vi "Car wash assignment.vi"() -> ()   [LabVIEW 2019]
panel:
  in  "Under Body Wash Position Switch":bool
  in  "Air Dry Position Switch":bool
  in  "Main Wash Position Switch":bool
  out "Wash Select":string
  out "Main wash TimeRemaining":dbl
  out "Main wash TimeElapsed":dbl
  out "Main wash":dbl
  out "Under/Air TimeRemaining":dbl
  out "Under/ Air TimeElapsed":dbl
  out "Under/Air":dbl
  in  "STOP":bool
  out "Vehicle Out of Position/\nPause":bool
  out "Air Dry":bool
  out "Clear Water Rinse":bool
  out "Main High Pressure Wash":bool
  out "Soap Application":bool
  out "Under Body Wash":bool
  in  "Economy Wash":bool
  in  "Deluxe Wash":bool
  out "Last Process":bool
  # "Purchase Selection"
  # "Car Wash Indicators"
  # "Car Wash Simulation Switches"
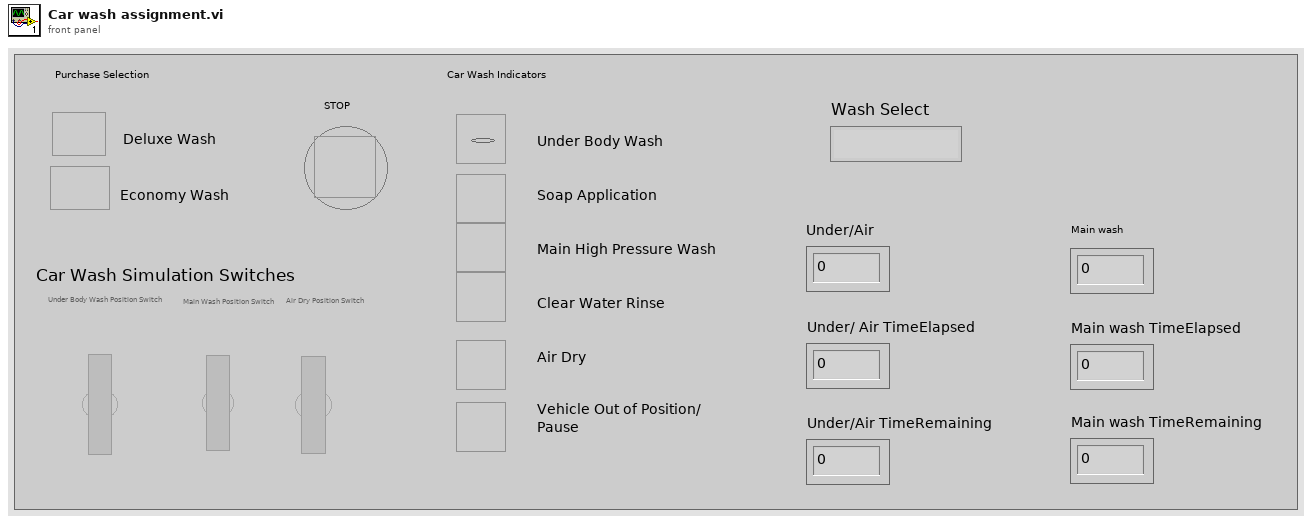
[diagram p1: front panel]
types:
  T1 = enum16{"Soap Application", "Pressure Wash", "CLear water rinse", "Vehicle out"}
  T2 = enum16{"Under Body Wash", "Soap Application", "Pressure Wash", "Clear Water Rinse", "Air Dry", "Vehicle out"}
  T3 = enum8{"Enabled", "Disabled", "Disabled and Grayed Out"}
  T4 = enum16{"Soap Application", "Pressure Wash", "Clear water rinse", "Vehicle out"}
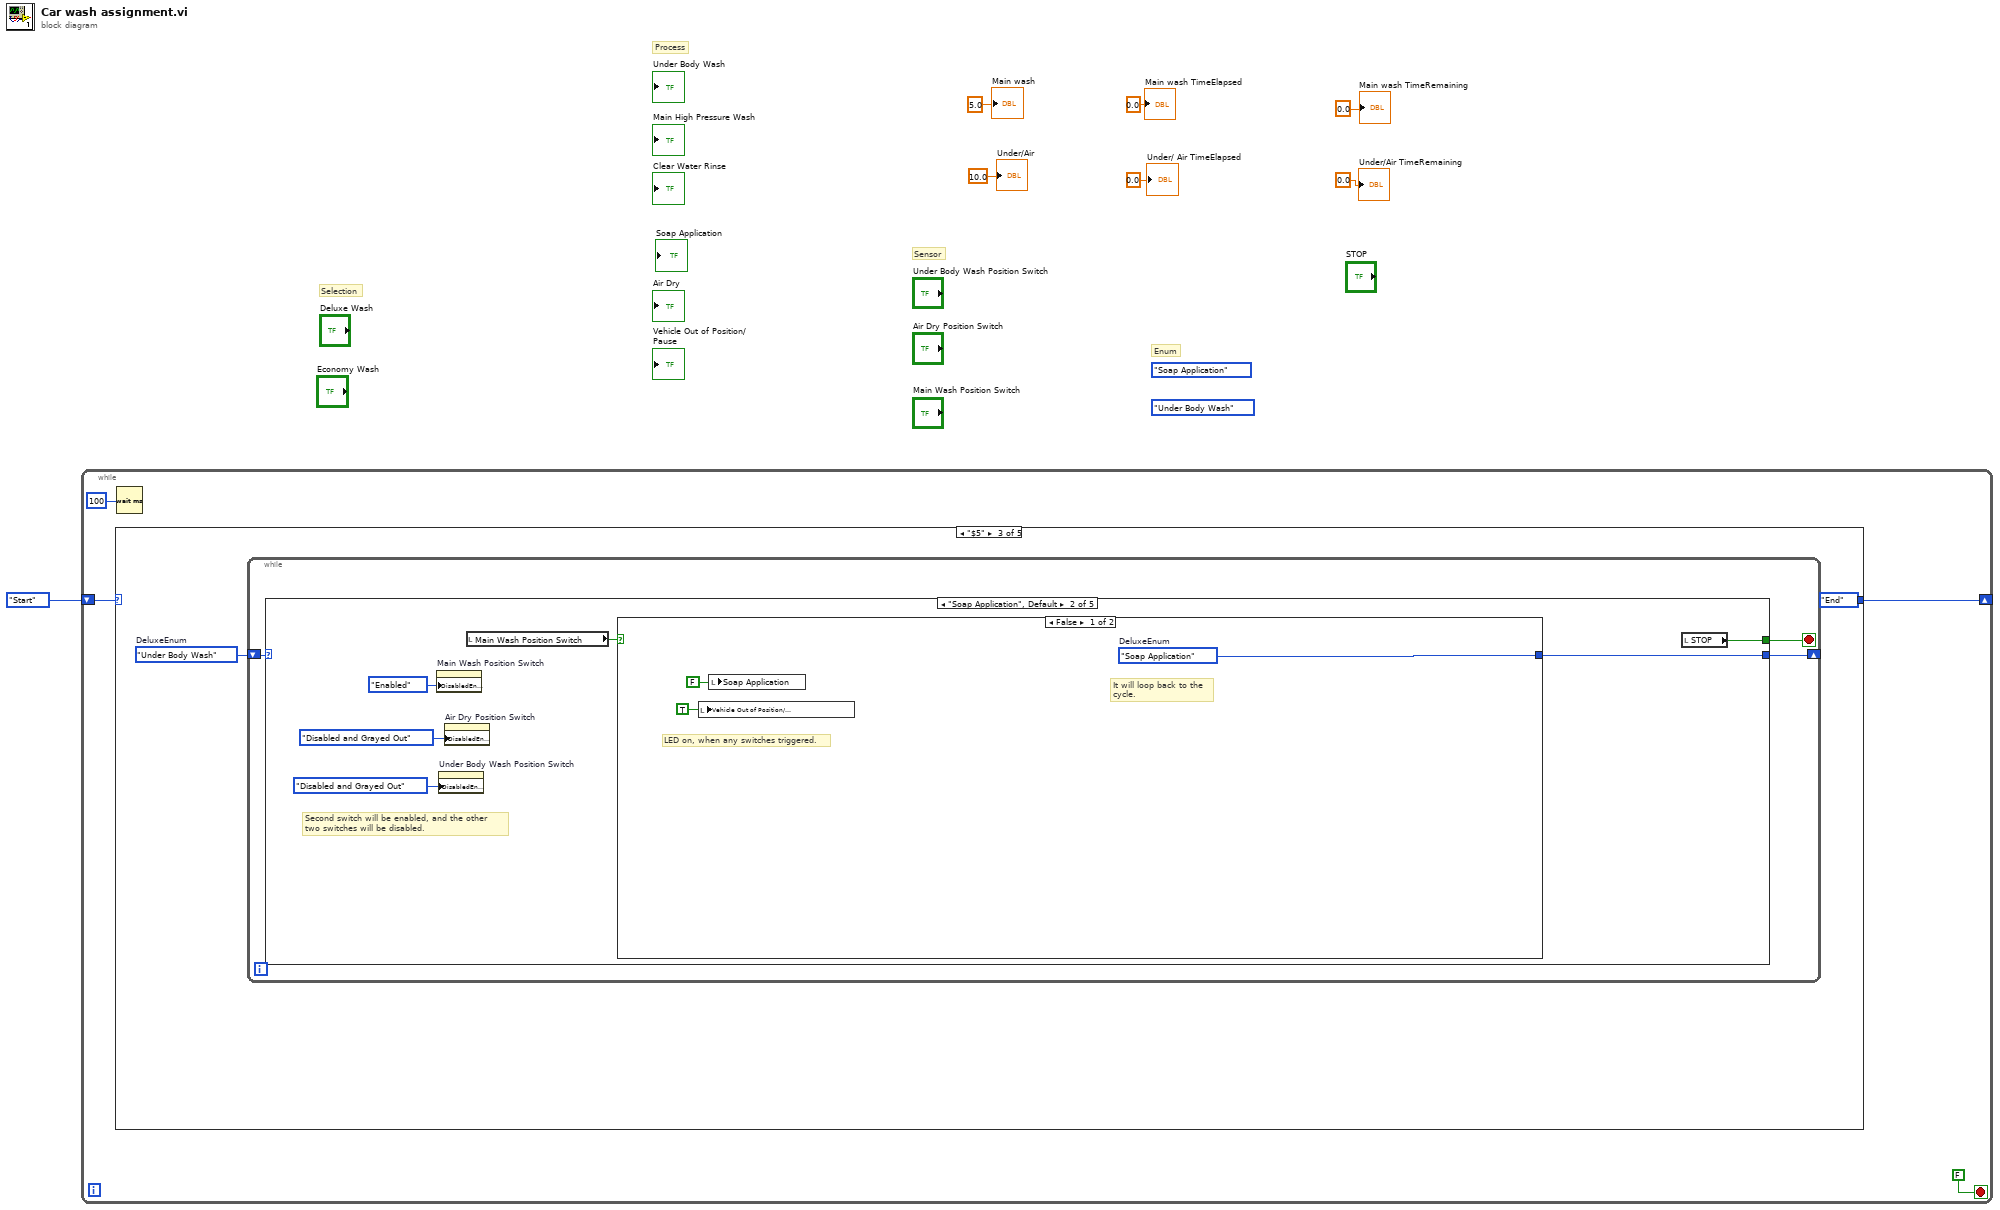
[diagram p0: block diagram]
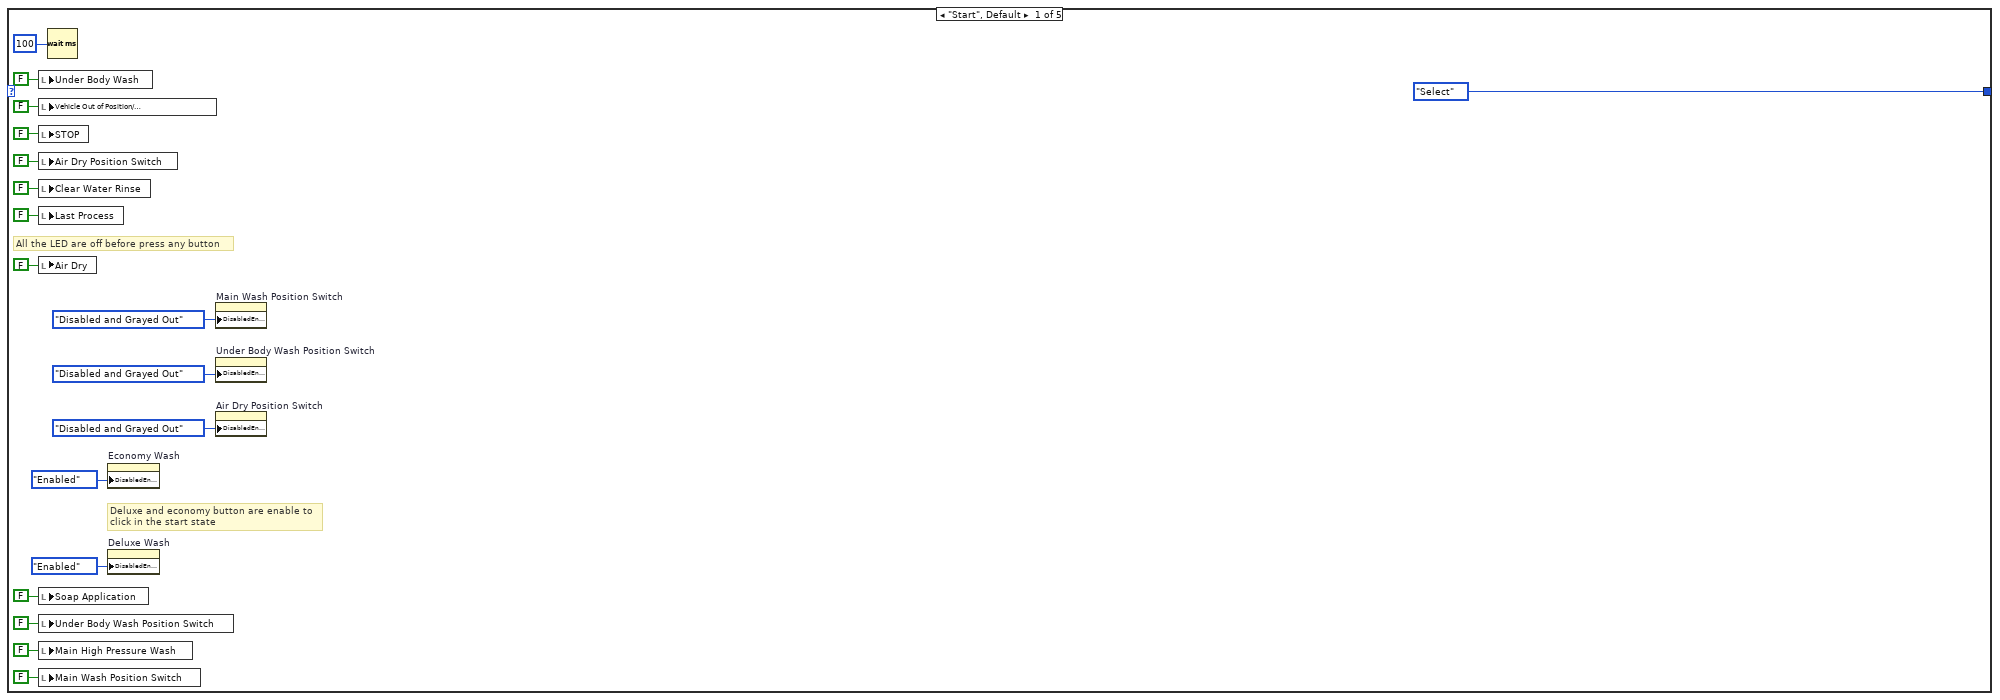
[diagram p2: hidden frame]
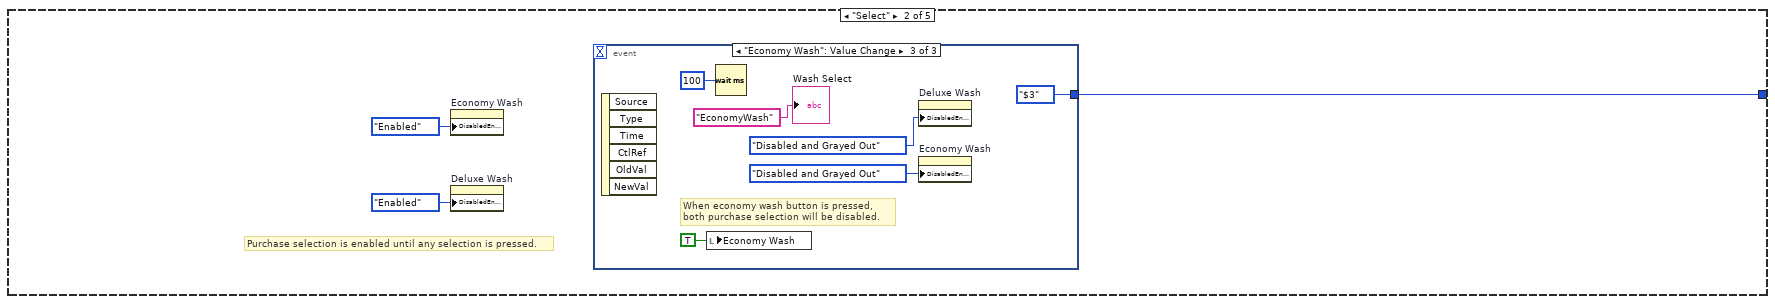
[diagram p3: hidden frame]
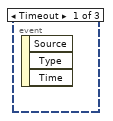
[diagram p4: hidden frame]
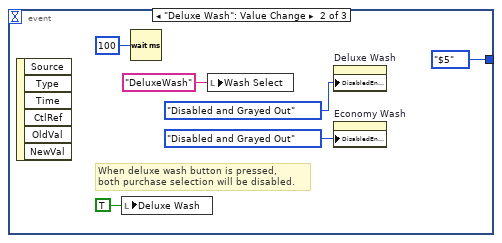
[diagram p5: hidden frame]
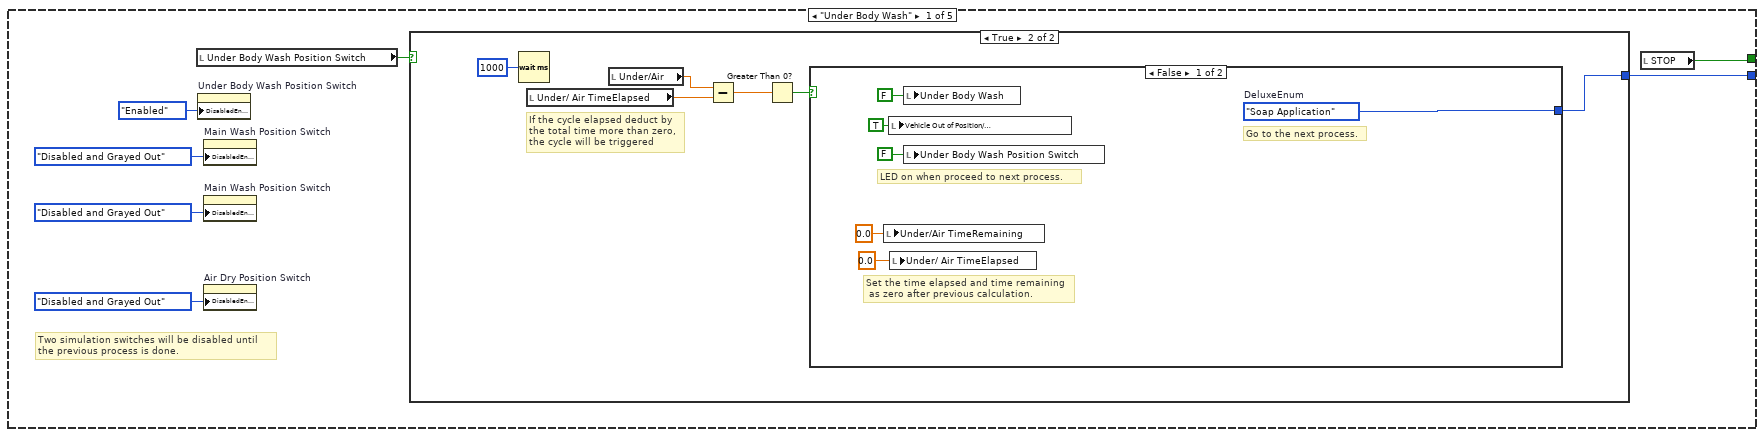
[diagram p6: hidden frame]
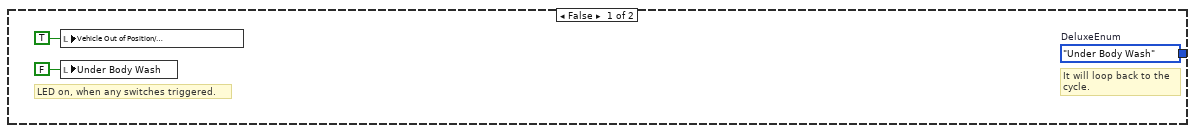
[diagram p7: hidden frame]
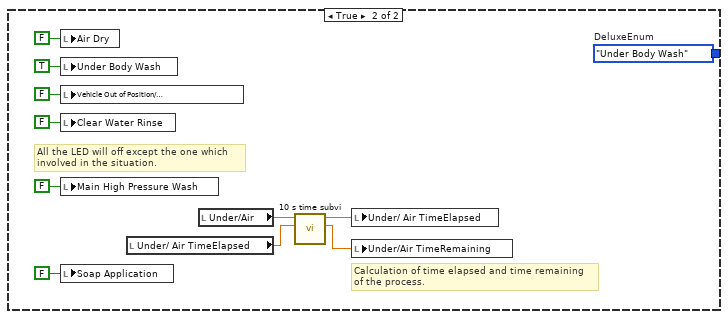
[diagram p8: hidden frame]
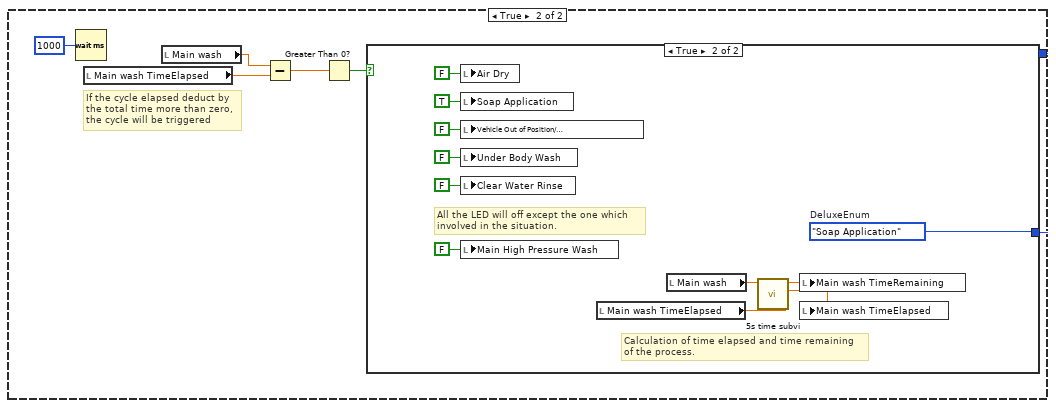
[diagram p9: hidden frame]
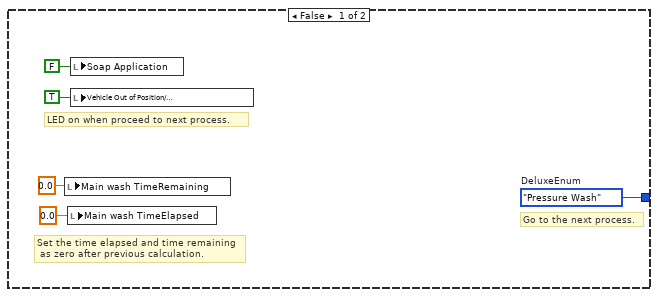
[diagram p10: hidden frame]
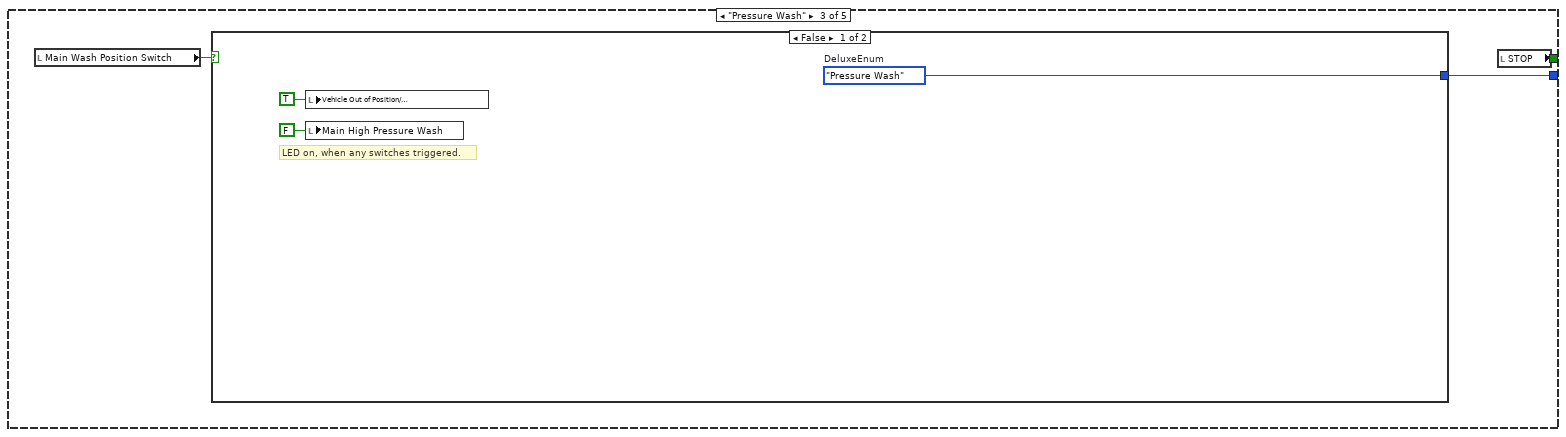
[diagram p11: hidden frame]
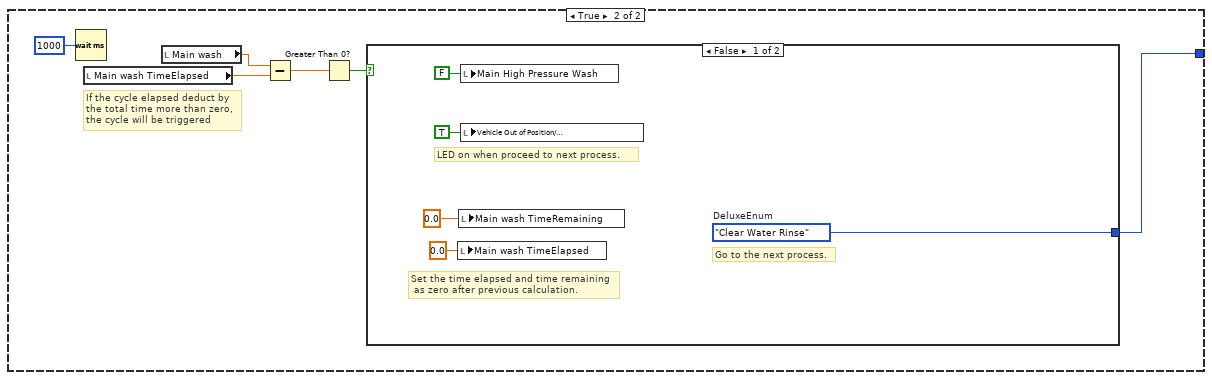
[diagram p12: hidden frame]
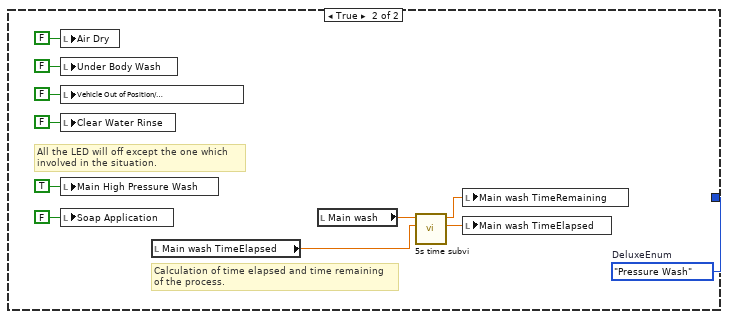
[diagram p13: hidden frame]
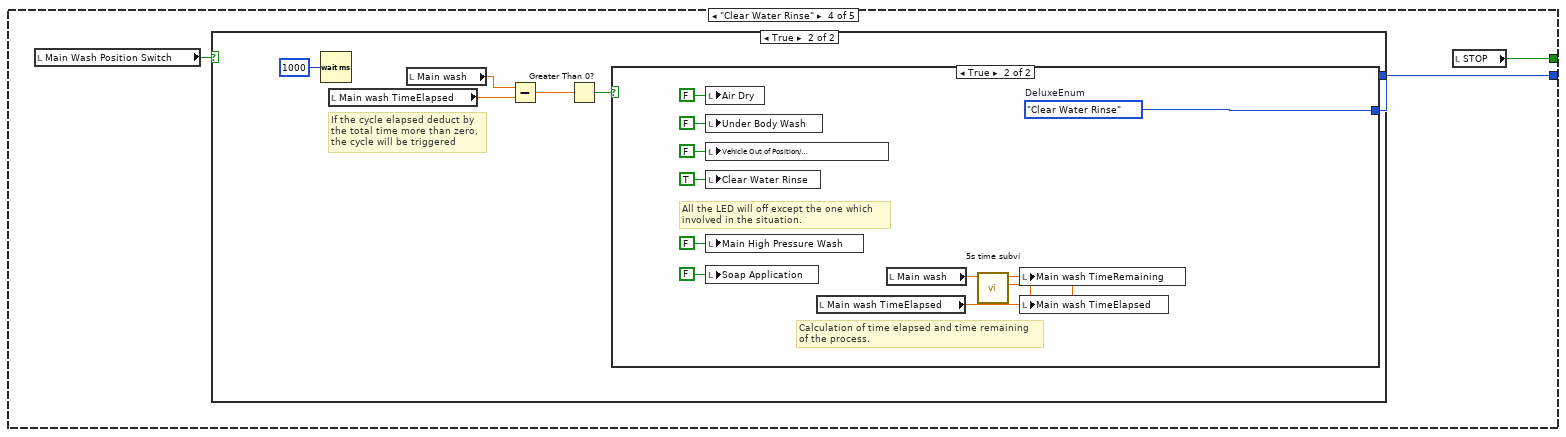
[diagram p14: hidden frame]
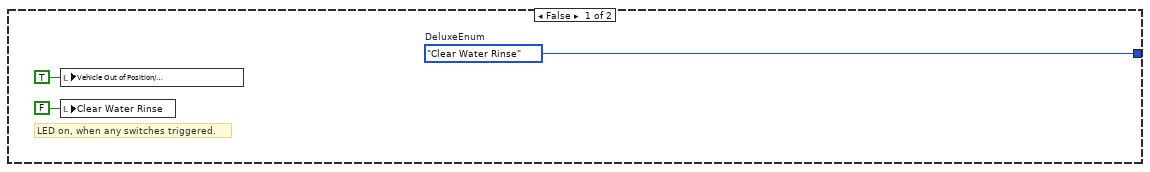
[diagram p15: hidden frame]
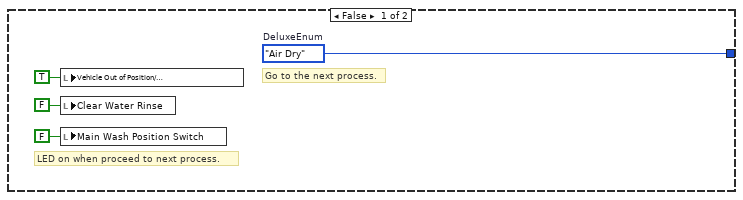
[diagram p16: hidden frame]
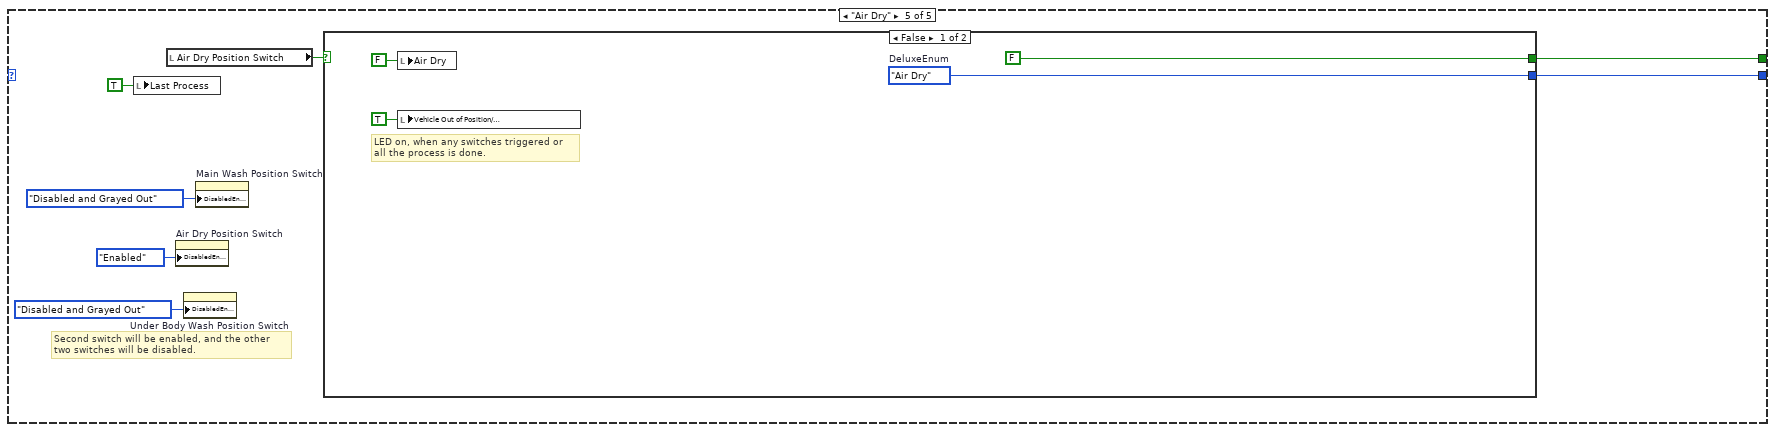
[diagram p17: hidden frame]
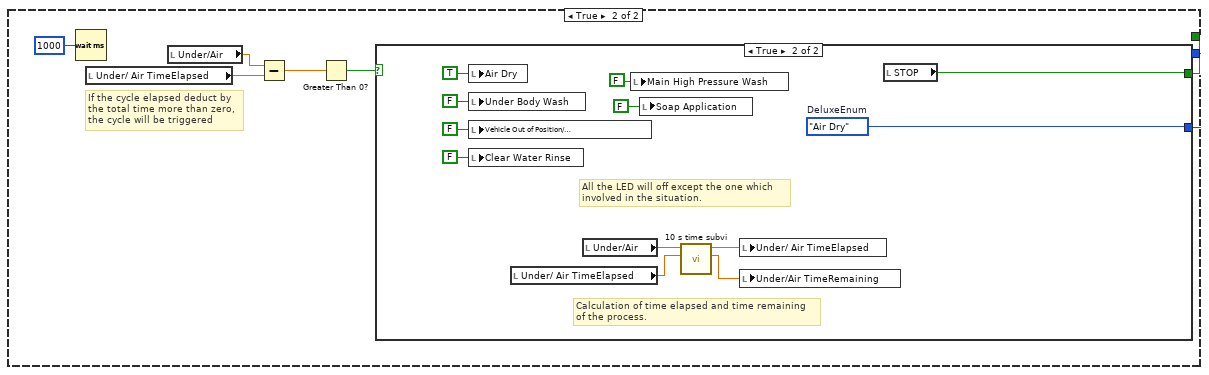
[diagram p18: hidden frame]
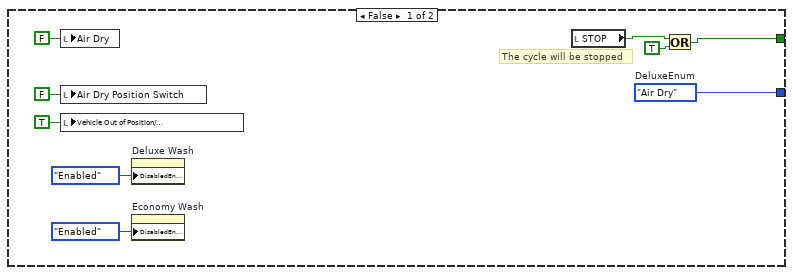
[diagram p19: hidden frame]
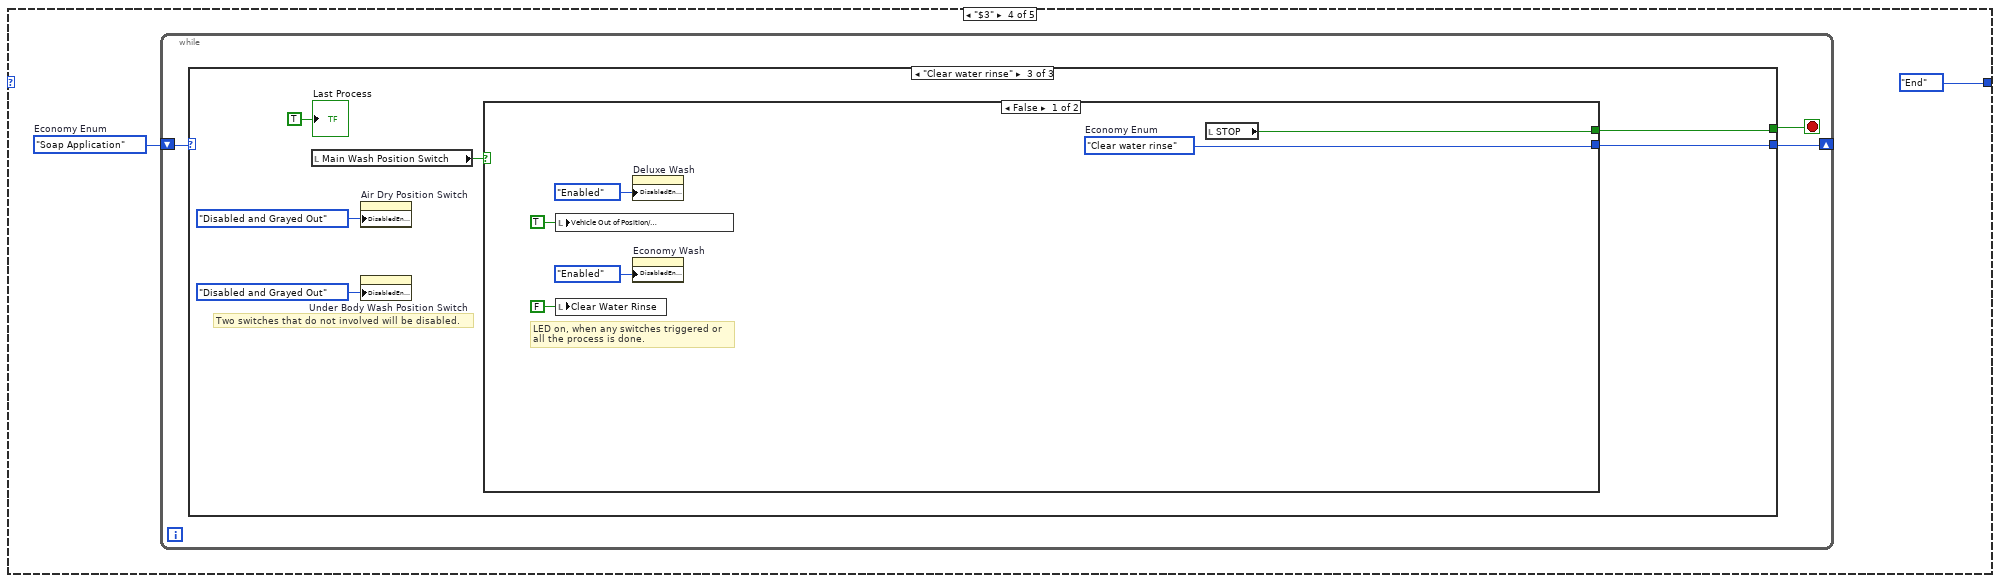
[diagram p20: hidden frame]
diagram:
  (unwired) T1."Soap Application" ("Economy Enum")
  (unwired) T2."Under Body Wash" ("Enum")
  # "Enum"
  # "Process"
  # "Sensor"
  # "Selection"
  n1 = while {
    shift-right: [w10] -> _
    shift-left: enum16{"Start", "Select", "$5", "$3", "End"}."Start" -> [w11]
    stop <- FALSE stop-if-true
    n2 = case shown="\"$5\"" w11 {
      tunnel: [enum16{"Start", "Select", "$5", "$3", "End"}."Select" w32 enum16{"Start", "Select", "$5", "$3", "End"}."End" enum16{"Start", "Select", "$5", "$3", "End"}."End" enum16{"Start", "Select", "$5", "$3", "End"}."Start"] -> w10
      frame "Start", Default {
        # "All the LED are off before press any button"
        # "Deluxe and economy button are enable to\nclick in the start state"
        n3 = local write "Under Body Wash"(FALSE ("Under Body Wash")) -> ()
        n4 = local write "Vehicle Out of Position/\nPause"(FALSE ("Vehicle Out of Position/\nPause")) -> ()
        n5 = local write "STOP"(FALSE ("STOP")) -> ()
        n6 = local write "Air Dry Position Switch"(FALSE ("Air Dry Position Switch")) -> ()
        n7 = local write "Clear Water Rinse"(FALSE ("Clear Water Rinse")) -> ()
        n8 = local write "Last Process"(FALSE ("Last Process")) -> ()
        n9 = local write "Air Dry"(FALSE ("Air Dry")) -> ()
        n10 = local write "Soap Application"(FALSE ("Soap Application")) -> ()
        n11 = local write "Under Body Wash Position Switch"(FALSE ("Under Body Wash Positition Switch")) -> ()
        n12 = local write "Main High Pressure Wash"(FALSE ("Main Hight Pressure Wash")) -> ()
        n13 = local write "Main Wash Position Switch"(FALSE ("Main Wash Position Switch")) -> ()
        n14 = Wait (ms)(milliseconds to wait=u32 100 ("millisecond timer value")) -> ()  [unwired: 1 out]
        n15 = property on="Economy Wash" class="Bool (strict)"("DisabledEnum"=T3."Enabled" ("Disabled")) -> ()  [unwired: 2 in, 2 out]
        n16 = property on="Deluxe Wash" class="Bool (strict)"("DisabledEnum"=T3."Enabled" ("Disabled")) -> ()  [unwired: 2 in, 2 out]
        n17 = property on="Main Wash Position Switch" class="Bool (strict)"("DisabledEnum"=T3."Disabled and Grayed Out" ("Disabled")) -> ()  [unwired: 2 in, 2 out]
        n18 = property on="Under Body Wash Position Switch" class="Bool (strict)"("DisabledEnum"=T3."Disabled and Grayed Out" ("Disabled")) -> ()  [unwired: 2 in, 2 out]
        n19 = property on="Air Dry Position Switch" class="Bool (strict)"("DisabledEnum"=T3."Disabled and Grayed Out" ("Disabled")) -> ()  [unwired: 2 in, 2 out]
      }
      frame "Select" {
        # "Purchase selection is enabled until any selection is pressed."
        n20 = property on="Economy Wash" class="Bool (strict)"("DisabledEnum"=T3."Enabled" ("Disabled")) -> ()  [unwired: 2 in, 2 out]
        n21 = property on="Deluxe Wash" class="Bool (strict)"("DisabledEnum"=T3."Enabled" ("Disabled")) -> ()  [unwired: 2 in, 2 out]
        n22 = event shown="[2] \"Economy Wash\": Value Change" {
          selector: _ -> [_ _ _]
          dyn-events: _ -> [_ _ _]
          timeout: _ -> [_ _ _]
          tunnel: [_ enum16{"Start", "Select", "$5", "$3", "End"}."$5" enum16{"Start", "Select", "$5", "$3", "End"}."$3"] -> w32
          event Timeout {
            n23 = event-data() -> ()  [unwired: 1 in, 3 out]
          }
          event "Deluxe Wash": Value Change {
            # "When deluxe wash button is pressed,\nboth purchase selection will be disabled."
            n24 = event-data() -> ()  [unwired: 1 in, 6 out]
            n25 = local write "Deluxe Wash"(TRUE ("Deluxe Wash")) -> ()
            n26 = Wait (ms)(milliseconds to wait=u32 100 ("millisecond timer value")) -> ()  [unwired: 1 out]
            n27 = local write "Wash Select"("DeluxeWash") -> ()
            n28 = property on="Deluxe Wash" class="Bool (strict)"("DisabledEnum"=T3."Disabled and Grayed Out" ("Disabled")) -> ()  [unwired: 2 in, 2 out]
            n29 = property on="Economy Wash" class="Bool (strict)"("DisabledEnum"=T3."Disabled and Grayed Out" ("Disabled")) -> ()  [unwired: 2 in, 2 out]
          }
          event "Economy Wash": Value Change {
            # "When economy wash button is pressed,\nboth purchase selection will be disabled."
            n30 = event-data() -> ()  [unwired: 1 in, 6 out]
            n31 = local write "Economy Wash"(TRUE ("Economy Wash")) -> ()
            n32 = Wait (ms)(milliseconds to wait=u32 100 ("millisecond timer value")) -> ()  [unwired: 1 out]
            n33 = property on="Deluxe Wash" class="Bool (strict)"("DisabledEnum"=T3."Disabled and Grayed Out" ("Disabled")) -> ()  [unwired: 2 in, 2 out]
            n34 = property on="Economy Wash" class="Bool (strict)"("DisabledEnum"=T3."Disabled and Grayed Out" ("Disabled")) -> ()  [unwired: 2 in, 2 out]
            "Wash Select" <- "EconomyWash"
          }
        }
      }
      frame "$5" {
        w45 = T2."Under Body Wash"  # DeluxeEnum
        n35 = while {
          shift-right: [w49] -> _
          shift-left: w45 -> [w48]
          stop <- w47 stop-if-true
          n36 = case shown="\"Soap Application\", Default" w48 {
            tunnel: [w55 w88 w115 w144 w174] -> w49
            tunnel: [w50 w83 w114 w142 w170] -> w47
            frame "Under Body Wash" {
              # "Two simulation switches will be disabled until\nthe previous process is done."
              n37 = local read "Under Body Wash Position Switch"() -> (w56:bool)
              n38 = property on="Under Body Wash Position Switch" class="Bool (strict)"("DisabledEnum"=T3."Enabled" ("Disabled")) -> ()  [unwired: 2 in, 2 out]
              n39 = property on="Main Wash Position Switch" class="Bool (strict)"("DisabledEnum"=T3."Disabled and Grayed Out" ("Disabled")) -> ()  [unwired: 2 in, 2 out]
              n40 = property on="Main Wash Position Switch" class="Bool (strict)"("DisabledEnum"=T3."Disabled and Grayed Out" ("Disabled")) -> ()  [unwired: 2 in, 2 out]
              n41 = property on="Air Dry Position Switch" class="Bool (strict)"("DisabledEnum"=T3."Disabled and Grayed Out" ("Disabled")) -> ()  [unwired: 2 in, 2 out]
              n42 = case shown="True" w56 {
                tunnel: [w57 w60] -> w55
                frame False {
                  w57 = T2."Under Body Wash"  # DeluxeEnum
                  # "LED on, when any switches triggered."
                  # "It will loop back to the\ncycle."
                  n43 = local write "Vehicle Out of Position/\nPause"(TRUE ("Vehicle Out of Position")) -> ()
                  n44 = local write "Under Body Wash"(FALSE ("Under Body Wash")) -> ()
                }
                frame True {
                  # "If the cycle elapsed deduct by \nthe total time more than zero,\nthe cycle will be triggered"
                  n45 = Wait (ms)(milliseconds to wait=u32 1000) -> ()  [unwired: 1 out]
                  n46 = local read "Under/ Air TimeElapsed"() -> (w63:dbl)
                  n47 = local read "Under/Air"() -> (w64:dbl)
                  n48 = Subtract(x=w64, y=w63) -> (x-y=w62:dbl)
                  n49 = Greater Than 0?(x=w62) -> (x > 0?=w61:bool)
                  n50 = case shown="False" w61 {
                    tunnel: [w71 w79] -> w60
                    frame False {
                      w71 = T2."Soap Application"  # DeluxeEnum
                      # "Go to the next process."
                      # "LED on when proceed to next process."
                      # "Set the time elapsed and time remaining\n as zero after previous calculation."
                      n51 = local write "Under/Air TimeRemaining"(0.0 ("Under/Air TimeRemaining")) -> ()
                      n52 = local write "Vehicle Out of Position/\nPause"(TRUE ("Vehicle Out of Position")) -> ()
                      n53 = local write "Under/ Air TimeElapsed"(0.0 ("Under/ Air TimeElapsed")) -> ()
                      n54 = local write "Under Body Wash"(FALSE ("Under Body Wash")) -> ()
                      n55 = local write "Under Body Wash Position Switch"(FALSE ("Under Body Wash Positition Switch")) -> ()
                    }
                    frame True {
                      w79 = T2."Under Body Wash"  # DeluxeEnum
                      # "Calculation of time elapsed and time remaining\nof the process."
                      # "All the LED will off except the one which\ninvolved in the situation."
                      n56 = local write "Air Dry"(FALSE ("Air Dry")) -> ()
                      n57 = local write "Under Body Wash"(TRUE ("Under Body Wash")) -> ()
                      n58 = local write "Vehicle Out of Position/\nPause"(FALSE ("Vehicle Out of Position")) -> ()
                      n59 = local write "Clear Water Rinse"(FALSE ("Clear Water Rinse")) -> ()
                      n60 = local write "Main High Pressure Wash"(FALSE ("Main Hight Pressure Wash")) -> ()
                      n61 = local write "Soap Application"(FALSE ("Soap Application")) -> ()
                      n62 = local read "Under/ Air TimeElapsed"() -> (w82:dbl)
                      n63 = local read "Under/Air"() -> (w81:dbl)
                      n64 = call "10 s time subvi.vi"("Under/ Air TimeElapsed"=w82, "Under/Air"=w81) -> ("Numeric 2"=w80:dbl, "Numeric"=w78:dbl)  [unwired: 8 in]
                      n65 = local write "Under/ Air TimeElapsed"(w78) -> ()
                      n66 = local write "Under/Air TimeRemaining"(w80) -> ()
                    }
                  }
                }
              }
              n67 = local read "STOP"() -> (w50:bool)
            }
            frame "Soap Application", Default {
              # "Second switch will be enabled, and the other \ntwo switches will be disabled."
              n68 = property on="Main Wash Position Switch" class="Bool (strict)"("DisabledEnum"=T3."Enabled" ("Disabled")) -> ()  [unwired: 2 in, 2 out]
              n69 = property on="Under Body Wash Position Switch" class="Bool (strict)"("DisabledEnum"=T3."Disabled and Grayed Out" ("Disabled")) -> ()  [unwired: 2 in, 2 out]
              n70 = property on="Air Dry Position Switch" class="Bool (strict)"("DisabledEnum"=T3."Disabled and Grayed Out" ("Disabled")) -> ()  [unwired: 2 in, 2 out]
              n71 = local read "Main Wash Position Switch"() -> (w87:bool)
              n72 = case shown="False" w87 {
                tunnel: [w89 w92] -> w88
                frame False {
                  w89 = T2."Soap Application"  # DeluxeEnum
                  # "It will loop back to the\ncycle."
                  # "LED on, when any switches triggered."
                  n73 = local write "Vehicle Out of Position/\nPause"(TRUE ("Vehicle Out of Position")) -> ()
                  n74 = local write "Soap Application"(FALSE ("Soap Application")) -> ()
                }
                frame True {
                  # "If the cycle elapsed deduct by \nthe total time more than zero,\nthe cycle will be triggered"
                  n75 = Wait (ms)(milliseconds to wait=u32 1000) -> ()  [unwired: 1 out]
                  n76 = local read "Main wash TimeElapsed"() -> (w93:dbl)
                  n77 = local read "Main wash"() -> (w94:dbl)
                  n78 = Subtract(x=w94, y=w93) -> (x-y=w96:dbl)
                  n79 = Greater Than 0?(x=w96) -> (x > 0?=w95:bool)
                  n80 = case shown="True" w95 {
                    tunnel: [w100 w113] -> w92
                    frame False {
                      w100 = T2."Pressure Wash"  # DeluxeEnum
                      # "Go to the next process."
                      # "LED on when proceed to next process."
                      # "Set the time elapsed and time remaining\n as zero after previous calculation."
                      n81 = local write "Main wash TimeRemaining"(0.0 ("Main wash TimeRemaining")) -> ()
                      n82 = local write "Main wash TimeElapsed"(0.0 ("Main wash TimeElapsed")) -> ()
                      n83 = local write "Soap Application"(FALSE ("Soap Application")) -> ()
                      n84 = local write "Vehicle Out of Position/\nPause"(TRUE ("Vehicle Out of Position")) -> ()
                    }
                    frame True {
                      w113 = T2."Soap Application"  # DeluxeEnum
                      # "All the LED will off except the one which\ninvolved in the situation."
                      # "Calculation of time elapsed and time remaining\nof the process."
                      n85 = local write "Air Dry"(FALSE ("Air Dry")) -> ()
                      n86 = local write "Soap Application"(TRUE ("Soap Application")) -> ()
                      n87 = local write "Vehicle Out of Position/\nPause"(FALSE ("Vehicle Out of Position")) -> ()
                      n88 = local write "Under Body Wash"(FALSE ("Under Body Wash")) -> ()
                      n89 = local write "Clear Water Rinse"(FALSE ("Clear Water Rinse")) -> ()
                      n90 = local write "Main High Pressure Wash"(FALSE ("Main Hight Pressure Wash")) -> ()
                      n91 = local read "Main wash TimeElapsed"() -> (w103:dbl)
                      n92 = local read "Main wash"() -> (w104:dbl)
                      n93 = call "5s time subvi.vi"("Main wash TimeElapsed"=w103, "Main wash"=w104) -> ("Numeric"=w105:dbl, "Numeric 2"=w106:dbl)  [unwired: 8 in]
                      n94 = local write "Main wash TimeRemaining"(w106) -> ()
                      n95 = local write "Main wash TimeElapsed"(w105) -> ()
                    }
                  }
                }
              }
              n96 = local read "STOP"() -> (w83:bool)
            }
            frame "Pressure Wash" {
              n97 = local read "Main Wash Position Switch"() -> (w116:bool)
              n98 = case shown="False" w116 {
                tunnel: [w117 w122] -> w115
                frame False {
                  w117 = T2."Pressure Wash"  # DeluxeEnum
                  # "LED on, when any switches triggered."
                  n99 = local write "Vehicle Out of Position/\nPause"(TRUE ("Vehicle Out of Position")) -> ()
                  n100 = local write "Main High Pressure Wash"(FALSE ("Main Hight Pressure Wash")) -> ()
                }
                frame True {
                  # "If the cycle elapsed deduct by \nthe total time more than zero,\nthe cycle will be triggered"
                  n101 = Wait (ms)(milliseconds to wait=u32 1000) -> ()  [unwired: 1 out]
                  n102 = local read "Main wash TimeElapsed"() -> (w120:dbl)
                  n103 = local read "Main wash"() -> (w121:dbl)
                  n104 = Subtract(x=w121, y=w120) -> (x-y=w124:dbl)
                  n105 = Greater Than 0?(x=w124) -> (x > 0?=w123:bool)
                  n106 = case shown="False" w123 {
                    tunnel: [w128 w141] -> w122
                    frame False {
                      w128 = T2."Clear Water Rinse"  # DeluxeEnum
                      # "Go to the next process."
                      # "LED on when proceed to next process."
                      # "Set the time elapsed and time remaining\n as zero after previous calculation."
                      n107 = local write "Main wash TimeElapsed"(0.0 ("Main wash TimeElapsed")) -> ()
                      n108 = local write "Main wash TimeRemaining"(0.0 ("Main wash TimeRemaining")) -> ()
                      n109 = local write "Main High Pressure Wash"(FALSE ("Main Hight Pressure Wash")) -> ()
                      n110 = local write "Vehicle Out of Position/\nPause"(TRUE ("Vehicle Out of Position")) -> ()
                    }
                    frame True {
                      w141 = T2."Pressure Wash"  # DeluxeEnum
                      # "All the LED will off except the one which\ninvolved in the situation."
                      # "Calculation of time elapsed and time remaining\nof the process."
                      n111 = local write "Air Dry"(FALSE ("Air Dry")) -> ()
                      n112 = local write "Under Body Wash"(FALSE ("Under Body Wash")) -> ()
                      n113 = local write "Vehicle Out of Position/\nPause"(FALSE ("Vehicle Out of Position")) -> ()
                      n114 = local write "Clear Water Rinse"(FALSE ("Clear Water Rinse")) -> ()
                      n115 = local write "Main High Pressure Wash"(TRUE ("Main Hight Pressure Wash")) -> ()
                      n116 = local write "Soap Application"(FALSE ("Soap Application")) -> ()
                      n117 = local read "Main wash TimeElapsed"() -> (w133:dbl)
                      n118 = local read "Main wash"() -> (w134:dbl)
                      n119 = call "5s time subvi.vi"("Main wash TimeElapsed"=w133, "Main wash"=w134) -> ("Numeric"=w131:dbl, "Numeric 2"=w132:dbl)  [unwired: 8 in]
                      n120 = local write "Main wash TimeRemaining"(w132) -> ()
                      n121 = local write "Main wash TimeElapsed"(w131) -> ()
                    }
                  }
                }
              }
              n122 = local read "STOP"() -> (w114:bool)
            }
            frame "Clear Water Rinse" {
              n123 = local read "Main Wash Position Switch"() -> (w143:bool)
              n124 = case shown="True" w143 {
                tunnel: [w145 w150] -> w144
                frame False {
                  w145 = T2."Clear Water Rinse"  # DeluxeEnum
                  # "LED on, when any switches triggered."
                  n125 = local write "Vehicle Out of Position/\nPause"(TRUE ("Vehicle Out of Position")) -> ()
                  n126 = local write "Clear Water Rinse"(FALSE ("Clear Water Rinse")) -> ()
                }
                frame True {
                  # "If the cycle elapsed deduct by \nthe total time more than zero,\nthe cycle will be triggered"
                  n127 = Wait (ms)(milliseconds to wait=u32 1000) -> ()  [unwired: 1 out]
                  n128 = local read "Main wash TimeElapsed"() -> (w148:dbl)
                  n129 = local read "Main wash"() -> (w149:dbl)
                  n130 = Subtract(x=w149, y=w148) -> (x-y=w152:dbl)
                  n131 = Greater Than 0?(x=w152) -> (x > 0?=w153:bool)
                  n132 = case shown="True" w153 {
                    tunnel: [w155 w168] -> w150
                    frame False {
                      w155 = T2."Air Dry"  # DeluxeEnum
                      # "Go to the next process."
                      # "LED on when proceed to next process."
                      n133 = local write "Vehicle Out of Position/\nPause"(TRUE ("Vehicle Out of Position")) -> ()
                      n134 = local write "Clear Water Rinse"(FALSE ("Clear Water Rinse")) -> ()
                      n135 = local write "Main Wash Position Switch"(FALSE ("Main Wash Position Switch")) -> ()
                    }
                    frame True {
                      w168 = T2."Clear Water Rinse"  # DeluxeEnum
                      # "All the LED will off except the one which\ninvolved in the situation."
                      # "Calculation of time elapsed and time remaining\nof the process."
                      n136 = local write "Air Dry"(FALSE ("Air Dry")) -> ()
                      n137 = local write "Under Body Wash"(FALSE ("Under Body Wash")) -> ()
                      n138 = local write "Vehicle Out of Position/\nPause"(FALSE ("Vehicle Out of Position")) -> ()
                      n139 = local write "Clear Water Rinse"(TRUE ("Clear Water Rinse")) -> ()
                      n140 = local write "Main High Pressure Wash"(FALSE ("Main Hight Pressure Wash")) -> ()
                      n141 = local write "Soap Application"(FALSE ("Soap Application")) -> ()
                      n142 = local read "Main wash TimeElapsed"() -> (w160:dbl)
                      n143 = local read "Main wash"() -> (w161:dbl)
                      n144 = call "5s time subvi.vi"("Main wash TimeElapsed"=w160, "Main wash"=w161) -> ("Numeric"=w158:dbl, "Numeric 2"=w159:dbl)  [unwired: 8 in]
                      n145 = local write "Main wash TimeRemaining"(w159) -> ()
                      n146 = local write "Main wash TimeElapsed"(w158) -> ()
                    }
                  }
                }
              }
              n147 = local read "STOP"() -> (w142:bool)
            }
            frame "Air Dry" {
              # "Second switch will be enabled, and the other \ntwo switches will be disabled."
              n148 = local write "Last Process"(TRUE ("Last Process")) -> ()
              n149 = local read "Air Dry Position Switch"() -> (w175:bool)
              n150 = property on="Air Dry Position Switch" class="Bool (strict)"("DisabledEnum"=T3."Enabled" ("Disabled")) -> ()  [unwired: 2 in, 2 out]
              n151 = property on="Under Body Wash Position Switch" class="Bool (strict)"("DisabledEnum"=T3."Disabled and Grayed Out" ("Disabled")) -> ()  [unwired: 2 in, 2 out]
              n152 = property on="Main Wash Position Switch" class="Bool (strict)"("DisabledEnum"=T3."Disabled and Grayed Out" ("Disabled")) -> ()  [unwired: 2 in, 2 out]
              n153 = case shown="False" w175 {
                tunnel: [w177 w183] -> w174
                tunnel: [FALSE w182] -> w170
                frame False {
                  w177 = T2."Air Dry"  # DeluxeEnum
                  # "LED on, when any switches triggered or\nall the process is done."
                  n154 = local write "Air Dry"(FALSE ("Air Dry")) -> ()
                  n155 = local write "Vehicle Out of Position/\nPause"(TRUE ("Vehicle Out of Position")) -> ()
                }
                frame True {
                  # "If the cycle elapsed deduct by \nthe total time more than zero,\nthe cycle will be triggered"
                  n156 = Wait (ms)(milliseconds to wait=u32 1000) -> ()  [unwired: 1 out]
                  n157 = local read "Under/ Air TimeElapsed"() -> (w180:dbl)
                  n158 = local read "Under/Air"() -> (w181:dbl)
                  n159 = Subtract(x=w181, y=w180) -> (x-y=w185:dbl)
                  n160 = Greater Than 0?(x=w185) -> (x > 0?=w186:bool)
                  n161 = case shown="True" w186 {
                    tunnel: [w193 w207] -> w183
                    tunnel: [w187 w196] -> w182
                    frame False {
                      w193 = T2."Air Dry"  # DeluxeEnum
                      # "The cycle will be stopped"
                      n162 = local write "Air Dry"(FALSE ("Air Dry")) -> ()
                      n163 = local write "Air Dry Position Switch"(FALSE ("Main Wash Position Switch")) -> ()
                      n164 = local write "Vehicle Out of Position/\nPause"(TRUE ("Vehicle Out of Position")) -> ()
                      n165 = property on="Deluxe Wash" class="Bool (strict)"("DisabledEnum"=T3."Enabled" ("Disabled")) -> ()  [unwired: 2 in, 2 out]
                      n166 = property on="Economy Wash" class="Bool (strict)"("DisabledEnum"=T3."Enabled" ("Disabled")) -> ()  [unwired: 2 in, 2 out]
                      n167 = local read "STOP"() -> (w188:bool)
                      n168 = Or(x=w188, y=TRUE ("x")) -> (x .or. y?=w187:bool)
                    }
                    frame True {
                      w207 = T2."Air Dry"  # DeluxeEnum
                      # "All the LED will off except the one which\ninvolved in the situation."
                      # "Calculation of time elapsed and time remaining\nof the process."
                      n169 = local write "Air Dry"(TRUE ("Air Dry")) -> ()
                      n170 = local write "Under Body Wash"(FALSE ("Under Body Wash")) -> ()
                      n171 = local write "Vehicle Out of Position/\nPause"(FALSE ("Vehicle Out of Position")) -> ()
                      n172 = local write "Clear Water Rinse"(FALSE ("Clear Water Rinse")) -> ()
                      n173 = local read "Under/ Air TimeElapsed"() -> (w200:dbl)
                      n174 = local read "Under/Air"() -> (w199:dbl)
                      n175 = local write "Main High Pressure Wash"(FALSE ("Main Hight Pressure Wash")) -> ()
                      n176 = local write "Soap Application"(FALSE ("Soap Application")) -> ()
                      n177 = call "10 s time subvi.vi"("Under/ Air TimeElapsed"=w200, "Under/Air"=w199) -> ("Numeric 2"=w198:dbl, "Numeric"=w197:dbl)  [unwired: 8 in]
                      n178 = local write "Under/ Air TimeElapsed"(w197) -> ()
                      n179 = local write "Under/Air TimeRemaining"(w198) -> ()
                      n180 = local read "STOP"() -> (w196:bool)
                    }
                  }
                }
              }
            }
          }
        }
      }
      frame "$3" {
        w208 = T4."Soap Application"  # Economy Enum
        n181 = while {
          shift-right: [w212] -> _
          shift-left: w208 -> [w211]
          stop <- w210 stop-if-true
          n182 = case shown="\"Clear water rinse\"" w211 {
            tunnel: [w218 w251 w283] -> w212
            tunnel: [w213 w248 w281] -> w210
            frame "Soap Application", Default {
              # "Two switches that do not involved will be disabled."
              n183 = local read "Main Wash Position Switch"() -> (w217:bool)
              n184 = property on="Main Wash Position Switch" class="Bool (strict)"("DisabledEnum"=T3."Enabled" ("Disabled")) -> ()  [unwired: 2 in, 2 out]
              n185 = property on="Air Dry Position Switch" class="Bool (strict)"("DisabledEnum"=T3."Disabled and Grayed Out" ("Disabled")) -> ()  [unwired: 2 in, 2 out]
              n186 = property on="Under Body Wash Position Switch" class="Bool (strict)"("DisabledEnum"=T3."Disabled and Grayed Out" ("Disabled")) -> ()  [unwired: 2 in, 2 out]
              n187 = case shown="False" w217 {
                tunnel: [w220 w226] -> w218
                tunnel: [FALSE ("STOP") w223] -> w213
                frame False {
                  w220 = T4."Soap Application"  # Economy Enum
                  # "LED on, when any switches triggered."
                  # "It will loop back to\nthe cycle."
                  n188 = local write "Vehicle Out of Position/\nPause"(TRUE ("Vehicle Out of Position")) -> ()
                  n189 = local write "Soap Application"(FALSE ("Soap Application")) -> ()
                }
                frame True {
                  # "If the cycle elapsed deduct by \nthe total time more than zero,\nthe cycle will be triggered"
                  n190 = Wait (ms)(milliseconds to wait=u32 1000) -> ()  [unwired: 1 out]
                  n191 = local read "Main wash TimeElapsed"() -> (w224:dbl)
                  n192 = local read "Main wash"() -> (w225:dbl)
                  n193 = Subtract(x=w225, y=w224) -> (x-y=w228:dbl)
                  n194 = Greater Than 0?(x=w228) -> (x > 0?=w227:bool)
                  n195 = case shown="False" w227 {
                    tunnel: [w233 w247] -> w226
                    tunnel: [w230 FALSE ("STOP")] -> w223
                    frame False {
                      w233 = T4."Pressure Wash"  # Economy Enum
                      # "go to the next process."
                      # "Set the time elapsed and time remaining\n as zero after previous calculation."
                      # "LED on when proceed to next process."
                      n196 = local write "Main wash TimeElapsed"(0.0 ("Main wash TimeElapsed")) -> ()
                      n197 = local write "Main wash TimeRemaining"(0.0 ("Main wash TimeRemaining")) -> ()
                      n198 = local write "Soap Application"(FALSE ("Soap Application")) -> ()
                      n199 = local write "Vehicle Out of Position/\nPause"(TRUE ("Vehicle Out of Position")) -> ()
                      n200 = local read "STOP"() -> (w230:bool)
                    }
                    frame True {
                      w247 = T4."Soap Application"  # Economy Enum
                      # "All the LED will off except the one which\ninvolved in the situation."
                      # "Calculation of time elapsed and time remaining\nof the process."
                      n201 = local write "Air Dry"(FALSE ("Air Dry")) -> ()
                      n202 = local write "Clear Water Rinse"(FALSE ("Clear Water Rinse")) -> ()
                      n203 = local write "Main High Pressure Wash"(FALSE ("Main Hight Pressure Wash")) -> ()
                      n204 = local write "Under Body Wash"(FALSE ("Under Body Wash")) -> ()
                      n205 = local write "Soap Application"(TRUE ("Soap Application")) -> ()
                      n206 = local write "Vehicle Out of Position/\nPause"(FALSE ("Vehicle Out of Position")) -> ()
                      n207 = local read "Main wash TimeElapsed"() -> (w239:dbl)
                      n208 = local read "Main wash"() -> (w240:dbl)
                      n209 = call "5s time subvi.vi"("Main wash TimeElapsed"=w239, "Main wash"=w240) -> ("Numeric"=w237:dbl, "Numeric 2"=w238:dbl)  [unwired: 8 in]
                      n210 = local write "Main wash TimeRemaining"(w238) -> ()
                      n211 = local write "Main wash TimeElapsed"(w237) -> ()
                    }
                  }
                }
              }
            }
            frame "Pressure Wash" {
              # "Two switches that do not involved will be disabled."
              n212 = local read "Main Wash Position Switch"() -> (w252:bool)
              n213 = property on="Under Body Wash Position Switch" class="Bool (strict)"("DisabledEnum"=T3."Disabled and Grayed Out" ("Disabled")) -> ()  [unwired: 2 in, 2 out]
              n214 = property on="Air Dry Position Switch" class="Bool (strict)"("DisabledEnum"=T3."Disabled and Grayed Out" ("Disabled")) -> ()  [unwired: 2 in, 2 out]
              n215 = case shown="True" w252 {
                tunnel: [w255 w258] -> w251
                frame False {
                  w255 = T4."Pressure Wash"  # Economy Enum
                  # "It will loop back to\nthe cycle."
                  # "LED on, when any switches triggered."
                  n216 = local write "Vehicle Out of Position/\nPause"(TRUE ("Vehicle Out of Position")) -> ()
                  n217 = local write "Clear Water Rinse"(FALSE ("Clear Water Rinse")) -> ()
                }
                frame True {
                  # "If the cycle elapsed deduct by \nthe total time more than zero,\nthe cycle will be triggered"
                  n218 = Wait (ms)(milliseconds to wait=u32 1000) -> ()  [unwired: 1 out]
                  n219 = local read "Main wash TimeElapsed"() -> (w256:dbl)
                  n220 = local read "Main wash"() -> (w257:dbl)
                  n221 = Subtract(x=w257, y=w256) -> (x-y=w261:dbl)
                  n222 = Greater Than 0?(x=w261) -> (x > 0?=w259:bool)
                  n223 = case shown="True" w259 {
                    tunnel: [w264 w277] -> w258
                    frame False {
                      w264 = T4."Clear water rinse"  # Economy Enum
                      # "go to the next process."
                      # "Set the time elapsed and time remaining\n as zero after previous calculation."
                      # "LED on when proceed to next process."
                      n224 = local write "Main wash TimeRemaining"(0.0 ("Main wash TimeRemaining")) -> ()
                      n225 = local write "Main High Pressure Wash"(FALSE ("Main Hight Pressure Wash")) -> ()
                      n226 = local write "Vehicle Out of Position/\nPause"(TRUE ("Vehicle Out of Position")) -> ()
                      n227 = local write "Main wash TimeElapsed"(0.0 ("Main wash TimeElapsed")) -> ()
                    }
                    frame True {
                      w277 = T4."Pressure Wash"  # Economy Enum
                      # "All the LED will off except the one which\ninvolved in the situation."
                      # "Calculation of time elapsed and time remaining\nof the process."
                      n228 = local write "Air Dry"(FALSE ("Air Dry")) -> ()
                      n229 = local write "Clear Water Rinse"(FALSE ("Clear Water Rinse")) -> ()
                      n230 = local write "Main High Pressure Wash"(TRUE ("Main Hight Pressure Wash")) -> ()
                      n231 = local write "Under Body Wash"(FALSE ("Under Body Wash")) -> ()
                      n232 = local write "Soap Application"(FALSE ("Soap Application")) -> ()
                      n233 = local write "Vehicle Out of Position/\nPause"(FALSE ("Vehicle Out of Position")) -> ()
                      n234 = local read "Main wash TimeElapsed"() -> (w269:dbl)
                      n235 = local read "Main wash"() -> (w270:dbl)
                      n236 = call "5s time subvi.vi"("Main wash TimeElapsed"=w269, "Main wash"=w270) -> ("Numeric"=w267:dbl, "Numeric 2"=w268:dbl)  [unwired: 8 in]
                      n237 = local write "Main wash TimeRemaining"(w268) -> ()
                      n238 = local write "Main wash TimeElapsed"(w267) -> ()
                    }
                  }
                }
              }
              n239 = local read "STOP"() -> (w248:bool)
            }
            frame "Clear water rinse" {
              # "Two switches that do not involved will be disabled."
              n240 = local read "Main Wash Position Switch"() -> (w282:bool)
              n241 = property on="Air Dry Position Switch" class="Bool (strict)"("DisabledEnum"=T3."Disabled and Grayed Out" ("Disabled")) -> ()  [unwired: 2 in, 2 out]
              n242 = property on="Under Body Wash Position Switch" class="Bool (strict)"("DisabledEnum"=T3."Disabled and Grayed Out" ("Disabled")) -> ()  [unwired: 2 in, 2 out]
              n243 = case shown="False" w282 {
                tunnel: [w287 w293] -> w283
                tunnel: [w284 w290] -> w281
                frame False {
                  w287 = T4."Clear water rinse"  # Economy Enum
                  # "LED on, when any switches triggered or \nall the process is done."
                  n244 = local write "Vehicle Out of Position/\nPause"(TRUE ("Vehicle Out of Position")) -> ()
                  n245 = local write "Clear Water Rinse"(FALSE ("Clear Water Rinse")) -> ()
                  n246 = property on="Deluxe Wash" class="Bool (strict)"("DisabledEnum"=T3."Enabled" ("Disabled")) -> ()  [unwired: 2 in, 2 out]
                  n247 = property on="Economy Wash" class="Bool (strict)"("DisabledEnum"=T3."Enabled" ("Disabled")) -> ()  [unwired: 2 in, 2 out]
                  n248 = local read "STOP"() -> (w284:bool)
                }
                frame True {
                  # "If the cycle elapsed deduct by \nthe total time more than zero,\nthe cycle will be triggered"
                  n249 = Wait (ms)(milliseconds to wait=u32 1000) -> ()  [unwired: 1 out]
                  n250 = local read "Main wash TimeElapsed"() -> (w291:dbl)
                  n251 = local read "Main wash"() -> (w292:dbl)
                  n252 = Subtract(x=w292, y=w291) -> (x-y=w296:dbl)
                  n253 = Greater Than 0?(x=w296) -> (x > 0?=w294:bool)
                  n254 = case shown="True" w294 {
                    tunnel: [w301 w315] -> w293
                    tunnel: [w297 w304] -> w290
                    frame False {
                      w301 = T4."Clear water rinse"  # Economy Enum
                      # "LED on when proceed to next process."
                      # "go to the next process"
                      n255 = local write "Vehicle Out of Position/\nPause"(TRUE ("Vehicle Out of Position")) -> ()
                      n256 = local write "Clear Water Rinse"(FALSE ("Clear Water Rinse")) -> ()
                      n257 = local write "Main Wash Position Switch"(FALSE ("Main Wash Position Switch")) -> ()
                      n258 = local read "STOP"() -> (w299:bool)
                      n259 = Or(x=w299, y=TRUE) -> (x .or. y?=w297:bool)
                    }
                    frame True {
                      w315 = T4."Clear water rinse"  # Economy Enum
                      # "It will loop back to \nthe cycle"
                      # "All the LED will off except the one which\ninvolved in the situation."
                      # "Calculation of time elapsed and time remaining\nof the process."
                      n260 = local read "Main wash TimeElapsed"() -> (w307:dbl)
                      n261 = local write "Air Dry"(FALSE ("Air Dry")) -> ()
                      n262 = local write "Clear Water Rinse"(TRUE ("Clear Water Rinse")) -> ()
                      n263 = local write "Main High Pressure Wash"(FALSE ("Main Hight Pressure Wash")) -> ()
                      n264 = local write "Under Body Wash"(FALSE ("Under Body Wash")) -> ()
                      n265 = local write "Soap Application"(FALSE ("Soap Application")) -> ()
                      n266 = local read "Main wash"() -> (w308:dbl)
                      n267 = call "5s time subvi.vi"("Main wash TimeElapsed"=w307, "Main wash"=w308) -> ("Numeric"=w305:dbl, "Numeric 2"=w306:dbl)  [unwired: 8 in]
                      n268 = local write "Main wash TimeRemaining"(w306) -> ()
                      n269 = local write "Main wash TimeElapsed"(w305) -> ()
                      n270 = local write "Vehicle Out of Position/\nPause"(FALSE ("Vehicle Out of Position")) -> ()
                      n271 = local read "STOP"() -> (w304:bool)
                    }
                  }
                }
              }
              "Last Process" <- TRUE ("Boolean")
            }
          }
        }
      }
      frame "End" {
        n272 = local read "Wash Select"() -> (w317:string)
        n273 = case shown="\"EconomyWash\", Default" w317 {
          tunnel: [w319 w324] -> w316
          frame "EconomyWash", Default {
            # "If time remaining euqal zero and\nit is the last process, then record in table."
            n274 = local read "Main wash TimeRemaining"() -> (w323:dbl)
            n275 = local read "Last Process"() -> (w320:bool)
            n276 = Equal?(x=w323, y=0.0) -> (x = y?=w321:bool)
            n277 = And(x=w321, y=w320) -> (x .and. y?=w319:bool)
          }
          frame "DeluxeWash" {
            n278 = local read "Under/Air TimeRemaining"() -> (w328:dbl)
            n279 = local read "Last Process"() -> (w326:bool)
            n280 = Equal?(x=w328, y=0.0) -> (x = y?=w327:bool)
            n281 = And(x=w327, y=w326) -> (x .and. y?=w324:bool)
          }
        }
        n282 = case shown="True" w316 {
          frame False {
          }
          frame True {
            w340 = u16 888  # remote port or service name
            w341 = 60000  # timeout ms (60000)
            w342 = enum16{"short", "long", "abbreviated"}."abbreviated"  # date format (0)
            # "write wash select"
            # "write time"
            # "convert to string"
            # "save string length"
            # "get byte of the data"
            # "Get current date and time"
            # "wash select"
            # "save time"
            # "write date"
            n283 = Get Date/Time String(date format (0)=w342) -> (date string=w337:string, time string=w334:string)  [unwired: 2 in]
            n284 = String Length(string=w337) -> (length=w339:i32)
            n285 = String Length(string=w334) -> (length=w336:i32)
            n286 = TCP Open Connection(remote port or service name=w340, timeout ms (60000)=w341) -> (connection ID=w347:refnum<k5>)  [unwired: 3 in, 1 out]
            n287 = Number To Decimal String(number=w339) -> (decimal integer string=w338:string)  [unwired: 1 in]
            n288 = local read "Wash Select"() -> (w329:string)
            n289 = Number To Decimal String(number=w336) -> (decimal integer string=w335:string)  [unwired: 1 in]
            n290 = String Length(string=w329) -> (length=w331:i32)
            n291 = TCP Write(connection ID=w347, data in=w338) -> (connection ID out=w346:refnum<k5>)  [unwired: 2 in, 2 out]
            n292 = TCP Write(connection ID=w346, data in=w337) -> (connection ID out=w345:refnum<k5>)  [unwired: 2 in, 2 out]
            n293 = Number To Decimal String(number=w331) -> (decimal integer string=w330:string)  [unwired: 1 in]
            n294 = TCP Write(connection ID=w345, data in=w335) -> (connection ID out=w344:refnum<k5>)  [unwired: 2 in, 2 out]
            n295 = TCP Write(connection ID=w344, data in=w334) -> (connection ID out=w343:refnum<k5>)  [unwired: 2 in, 2 out]
            n296 = TCP Write(connection ID=w343, data in=w330) -> (connection ID out=w333:refnum<k5>)  [unwired: 2 in, 2 out]
            n297 = TCP Write(connection ID=w333, data in=w329) -> (connection ID out=w332:refnum<k5>)  [unwired: 2 in, 2 out]
            n298 = TCP Close Connection(connection ID=w332) -> ()  [unwired: 2 in, 2 out]
          }
        }
      }
    }
    n299 = Wait (ms)(milliseconds to wait=u32 100 ("millisecond timer value")) -> ()  [unwired: 1 out]
  }
  "Under/Air" <- 10.0 ("UnderBodyWash")
  "Under/ Air TimeElapsed" <- 0.0 ("UnderTimeElapsed")
  "Under/Air TimeRemaining" <- 0.0 ("UnderTimeRemaining")
  "Main wash" <- 5.0 ("SoapApplication")
  "Main wash TimeElapsed" <- 0.0 ("SoapTimeElapsed")
  "Main wash TimeRemaining" <- 0.0 ("SoapTimeRemaining")
